vi "niDTS WLAN DUT TEST state changes.vi"(8 "error in (no error)":errorcluster, 11 "niDTS WLAN DUT in":refnum<class "niDTS WLAN Dut.lvclass">) -> (0 "error out":errorcluster, 3 "niDTS WLAN DUT out":refnum<class "niDTS WLAN Dut.lvclass">)   [LabVIEW 2015, in "niDTS WLAN.lvlib" / "niDTS WLAN Dut.lvclass"]
uses:
  niDTS WLAN Dut.lvclass
panel:
  out "State Change:WLAN Type Changed":bool
  out "State Change:Standard Changed":bool
  out "State Change:Power Changed":bool
  out "State Change:OFDM Data Rate Changed":bool
  out "State Change:N Spatial Streams Changed":bool
  out "State Change:N Chains Changed":bool
  out "State Change:MCS Index Changed":bool
  out "State Change:Guard Interval Changed":bool
  out "State Change:Frequency Changed":bool
  out "State Change:FEC Coding Changed":bool
  out "State Change:DSSS Data Rate Changed":bool
  out "State Change:Channel Changed":bool
  out "State Change:Chains Changed":bool
  out "State Change:Bandwidth Changed":bool
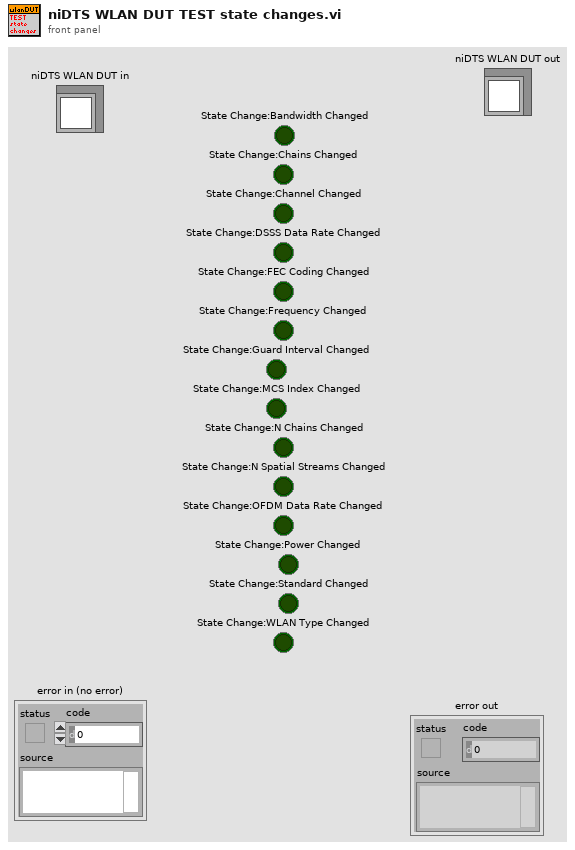
[diagram p1: front panel]
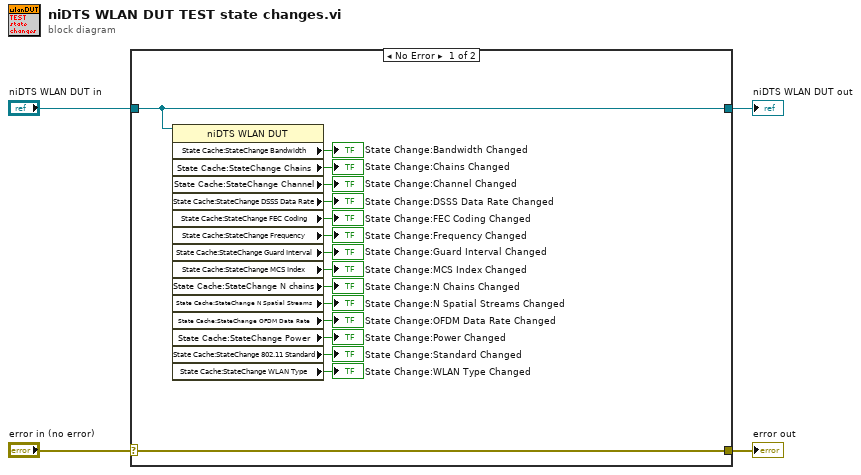
[diagram p0: block diagram]
diagram:
  n1 = case shown="No Error" "error in (no error)" {
    selector: "error in (no error)" -> [w20 w22]
    tunnel: [w20 w22] -> w3
    tunnel: [w19 w21] -> w1
    tunnel: "niDTS WLAN DUT in" -> [w19 w21]
    frame No Error {
      n2 = property class="niDTS WLAN DUT"(reference=w19) -> ("State Cache:StateChange Bandwidth"=→"State Change:Bandwidth Changed":bool, "State Cache:StateChange Chains"=→"State Change:Chains Changed":bool, "State Cache:StateChange Channel"=→"State Change:Channel Changed":bool, "State Cache:StateChange DSSS Data Rate"=→"State Change:DSSS Data Rate Changed":bool, "State Cache:StateChange FEC Coding"=→"State Change:FEC Coding Changed":bool, "State Cache:StateChange Frequency"=→"State Change:Frequency Changed":bool, "State Cache:StateChange Guard Interval"=→"State Change:Guard Interval Changed":bool, "State Cache:StateChange MCS Index"=→"State Change:MCS Index Changed":bool, "State Cache:StateChange N chains"=→"State Change:N Chains Changed":bool, "State Cache:StateChange N Spatial Streams"=→"State Change:N Spatial Streams Changed":bool, "State Cache:StateChange OFDM Data Rate"=→"State Change:OFDM Data Rate Changed":bool, "State Cache:StateChange Power"=→"State Change:Power Changed":bool, "State Cache:StateChange 802.11 Standard"=→"State Change:Standard Changed":bool, "State Cache:StateChange WLAN Type"=→"State Change:WLAN Type Changed":bool)  [unwired: 1 in, 2 out]
    }
    frame Error {
    }
  }
  "error out" <- w3
  "niDTS WLAN DUT out" <- w1
